vi "Execute.vi"(8 "error in":errorcluster, 11 "O3 Valve Step in":refnum<class "UV Power Step.lvclass">) -> (0 "error out":errorcluster, 1 "Next Step?":bool, 2 "MSG":string, 3 "O3 Valve Step out":refnum<class "UV Power Step.lvclass">)   [LabVIEW 2016, in "Controller.lvlib" / "UV Power Step.lvclass"]
uses:
  UV Power Step.lvclass
  C:/Program Files (x86)/National Instruments/LabVIEW 2016/vi.lib/MSR Consulting, LLC/General Reuse/Sequence/STEPS/LEAVES/Switch/Switch Step.lvclass
  Messages/Update UV Lamp State MSG/Update UV Lamp State MSG.lvclass
  G:/sw_repo/For Builds/Nicholas/Controller/Messages/Generic Boolean MSG/Generic Boolean Message.lvclass
  C:/Program Files (x86)/National Instruments/LabVIEW 2016/vi.lib/ActorFramework/Message/Message.lvclass
  Messages/Generic Boolean MSG/Generic Boolean Message.lvclass/Generic Boolean Message.ctl
  <vilib>/ActorFramework/Message Enqueuer/Message Enqueuer.lvclass/Message Enqueuer.ctl
  Messages/Generic Boolean MSG/Write Bool.vi
  <vilib>/ActorFramework/Message Priority Queue/Priority Enqueue.vi
  gController.lvclass
  <vilib>/ActorFramework/Message Enqueuer/Message Enqueuer.lvclass
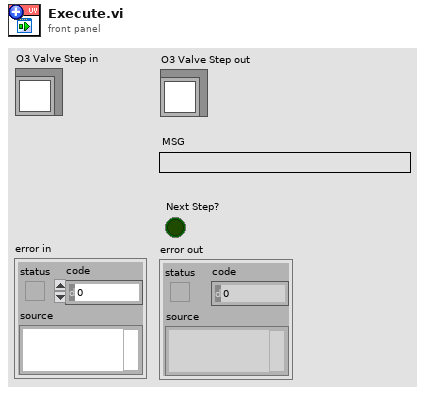
[diagram p1: front panel]
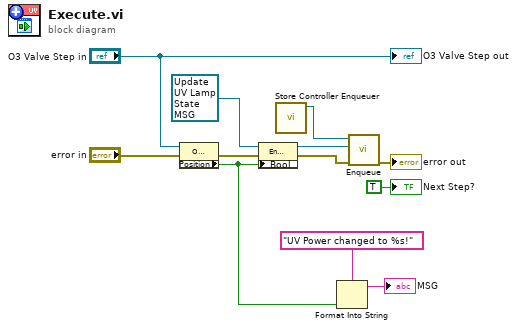
[diagram p0: block diagram]
diagram:
  n1 = property class="O2 Valve Step"(reference="O3 Valve Step in", error in="error in") -> (error out=w8:errorcluster, "Position"=w3:bool)  [unwired: 1 out]
  n2 = property class="Enable UV Lamp MSG"(reference=refnum<class "Update UV Lamp State MSG.lvclass"> refnum ("Controller.lvlib:Enable UV Lamp MSG"), error in=w8, "Bool"=w3) -> (reference out=w11:refnum<class "Update UV Lamp State MSG.lvclass">, error out=w7:errorcluster)
  n3 = call "Store Controller Enqueuer.vi"() -> ("Controller Enqueuer Out"=w12:refnum<class "Message Enqueuer.lvclass">)  [unwired: 11 in]
  n4 = Format Into String(format string="UV Power changed to %s!" ("MSG 2"), w3) -> (resulting string=→"MSG":string)  [unwired: 2 in, 1 out]
  n5 = call <vilib>:"Enqueue.vi"("error in (no error)"=w7, "Message"=w11, "Message Enqueuer in"=w12) -> ("error out"=→"error out":errorcluster)  [unwired: 7 in, 1 out]
  "O3 Valve Step out" <- "O3 Valve Step in"
  "Next Step?" <- TRUE ("Next Step?")
